vi "Configure Scan.vi"(0 "VISA resource name":refnum<visa-resource-name>, 1 "Channel List (101:110)":string, 7 "Sample Count (100)":i32=100, 11 "error in (no error)":errorcluster) -> (4 "VISA resource name out":refnum<visa-resource-name>, 15 "error out":errorcluster)   [LabVIEW 2013, in "Keithley 27XX.lvlib"]
doc: "This VI configures the channel list and sample size. It also enables the scan list for the next measurement. Use the Disable Scan.vi to disable the scan.\n\nIf the channel list is empty, the channel list will be ignored and the scan will not be enabled. the only setting which will be configured is the Sample Count."
uses:
  <instrlib>/Keithley 27XX/Keithley 27XX.lvlib
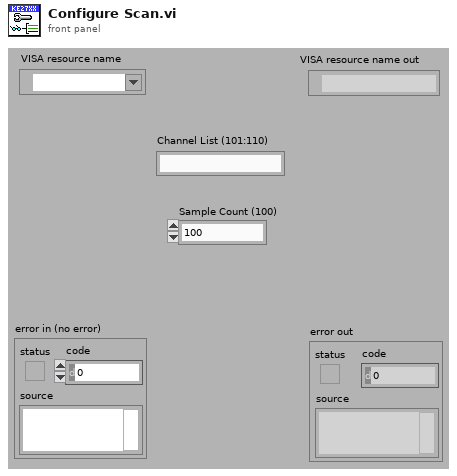
[diagram p1: front panel]
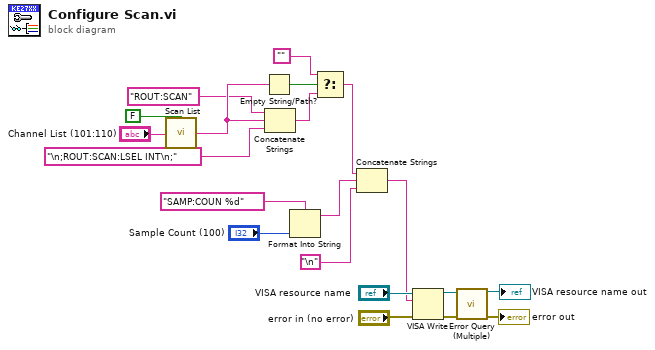
[diagram p0: block diagram]
diagram:
  n1 = call <instrlib>:"Scan List.vi"("Add Comma (True)"=FALSE ("Comma? (True)"), "Scan List (Empty)"="Channel List (101:110)") -> ("Scan List Out"=w20:string)  [unwired: 13 in]
  n2 = Empty String/Path?(string/path=w20) -> (empty?=w4:bool)
  n3 = Concatenate Strings("ROUT:SCAN", w20, "\n;ROUT:SCAN:LSEL INT\n;" ("string (\"\")")) -> (w1:string)
  n4 = Format Into String(format string="SAMP:COUN %d" ("string (\"\")"), "Sample Count (100)") -> (resulting string=w7:string)  [unwired: 2 in, 1 out]
  n5 = Select(t="", s=w4, f=w1) -> (s? t:f=w3:string)
  n6 = Concatenate Strings(w3, w7, "\n") -> (w16:string)
  n7 = VISA Write(VISA resource name="VISA resource name", write buffer=w16, error in (no error)="error in (no error)") -> (VISA resource name out=w13:refnum<visa-resource-name>, error out=w12:errorcluster)  [unwired: 1 out]
  n8 = call <instrlib>:"Error Query (Multiple).vi"("VISA resource name"=w13, "error in (no error)"=w12) -> ("VISA resource name out"=→"VISA resource name out":refnum<visa-resource-name>, "error out"=→"error out":errorcluster)  [unwired: 10 in, 2 out]
